vi "read default menu name.vi"(8 "error in":errorcluster, 11 "Targets in":refnum<class "Targets.lvclass">) -> (0 "error out":errorcluster, 2 "default menu name":string, 3 "Targets out":refnum<class "Targets.lvclass">)   [LabVIEW 2013, in "PL Framework Configuration Tool.lvlib" / "Targets.lvclass"]
uses:
  Targets.lvclass
  Framework Configuration Classes/target configuration/PL_Target Configuration.lvclass
  Framework Configuration Classes/target configuration/PL_Target Configuration.lvclass/PL_Target Configuration.ctl
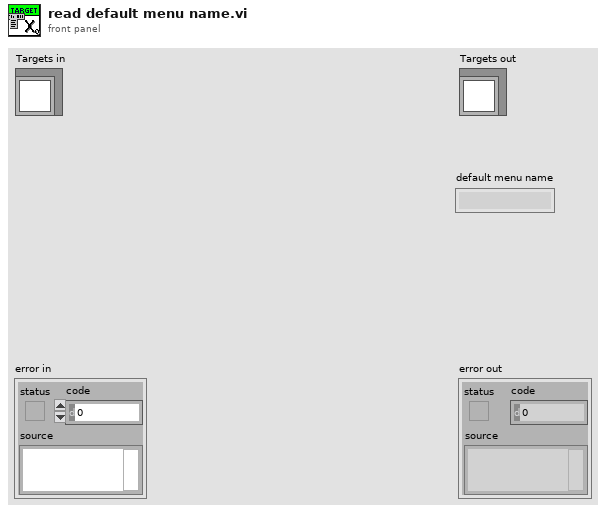
[diagram p1: front panel]
types:
  T1 = typedef "TBM configuration.lvclass/Target Types.ctl" = enum16{"Windows", "Mac", "Linux", "Linux RT ARM", "VxWorks", "Pharlap", "Other", "Linux RT x64"}
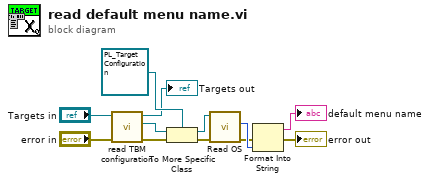
[diagram p0: block diagram]
diagram:
  n1 = call-dynamic "read TBM configuration.vi"("error in"="error in", "TBM Configuration Node in"="Targets in") -> ("error out"=w10:errorcluster, "configuration"=w11:refnum<class "TBM configuration.lvclass">, "TBM Configuration Node out"=→"Targets out":refnum<class "Targets.lvclass">)  [unwired: 7 in]
  n2 = To More Specific Class(target class=refnum<class "PL_Target Configuration.lvclass"> refnum ("Target Configuration"), reference=w11, error in=w10) -> (specific class reference=w8:refnum<class "PL_Target Configuration.lvclass">, error out=w9:errorcluster)
  n3 = call "Read OS.vi"("error in"=w9, "PL_Target Configuration in"=w8) -> ("error out"=w6:errorcluster, "Target Types"=w7:T1)  [unwired: 7 in, 1 out]
  n4 = Format Into String(error in=w6, w7) -> (resulting string=→"default menu name":string, error out=→"error out":errorcluster)  [unwired: 2 in]
